vi "Delete Timeout.vi"(0 "State in":refnum<class "State.lvclass">, 7 "termIndex":i32, 11 "error in (no error)":errorcluster) -> (4 "State out":refnum<class "State.lvclass">, 15 "error out":errorcluster)   [LabVIEW 2015, in "State.lvclass"]
uses:
  State.lvclass
  State.lvclass/State.ctl
  Timeout/Timeout.lvclass/Timeout.ctl
  Timeout/Write Link to.vi
  Timeout/Read Type.vi
  Timeout/Timeout.lvclass
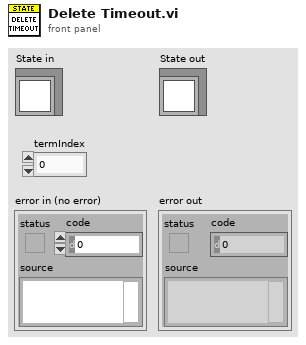
[diagram p1: front panel]
types:
  T1 = typedef "Tosca-Event Type.ctl" = enum16{"Normal", "CS+", "CS-"}
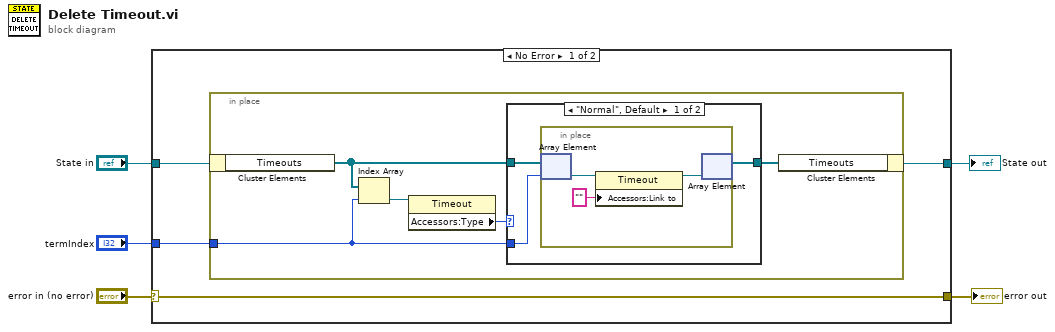
[diagram p0: block diagram]
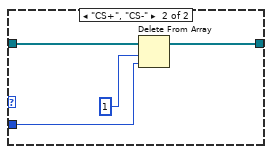
[diagram p2: hidden frame]
diagram:
  n1 = case shown="No Error" "error in (no error)" {
    selector: "error in (no error)" -> [w9 w26]
    tunnel: [w9 w26] -> w4
    tunnel: "State in" -> [w8 w25]
    tunnel: "termIndex" -> [w7 _]
    tunnel: [w6 w25] -> w1
    frame No Error {
      n2 = in-place {
        in-place-border: w7 -> [w12]
        n3 = in-place-cluster #1(w8) -> ("Timeouts"=w13:refnum<class "Timeout.lvclass">[])
        n4 = Index Array(array=w13, index=w12) -> (element=w11:refnum<class "Timeout.lvclass">)
        n5 = property class="Timeout"(reference=w11) -> ("Accessors:Type"=w10:T1)  [unwired: 1 in, 2 out]
        n6 = case shown="\"Normal\", Default" w10 {
          tunnel: [w15 w23] -> w14
          tunnel: w13 -> [w17 w22]
          tunnel: w12 -> [w16 w21]
          frame "Normal", Default {
            n7 = in-place {
              n8 = in-place-array #2(w17, w16) -> (w20:refnum<class "Timeout.lvclass">)
              n9 = property class="Timeout"(reference=w20, "Accessors:Link to"="" ("Link to")) -> (reference out=w19:refnum<class "Timeout.lvclass">)  [unwired: 1 in, 1 out]
              n10 = in-place-array #2(w19) -> (w15:refnum<class "Timeout.lvclass">[])  [unwired: 1 out]
            }
          }
          frame "CS+", "CS-" {
            n11 = Delete From Array(array=w22, length=1, index=w21) -> (array with subset deleted=w23:refnum<class "Timeout.lvclass">[])  [unwired: 1 out]
          }
        }
        n12 = in-place-cluster #1("Timeouts"=w14) -> (w6:refnum<class "State.lvclass">)
      }
    }
    frame Error {
    }
  }
  "error out" <- w4
  "State out" <- w1
